vi "PCO_SetFrameRate.vi"(0 "ph":u64, 5 "wFrameRateMode":u16, 7 "dwFrameRate":u32, 9 "dwFrameRateExposure":u32, 11 "error in (no error)":errorcluster {"code" format="%x"}) -> (3 "wFrameRateStatus":u16, 4 "ph out":u64, 6 "ErrorMessage":i32 format="%x", 8 "dwFrameRate out":u32, 10 "dwFrameRateExposure out":u32, 15 "error out":errorcluster {"code" format="%x"})   [LabVIEW 2019, in "SDK.lvlib" / "TimingControl.lvlib"]
doc: "<b>Description:</b>\nThis function does directly set the frame rate and the exposure time of the camera. The frame rate is limited by the readout time and the exposure time.\n\nframe rate <= 1/t_readout frame rate <= 1/t_expos\n\nPlease note that there are some overhead times, therefore the real values can differ slightly, e.g. the maximum frame rate will be a little bit less than 1 / exposure time. The in wFramerateMode parameter defines how the function works if any of the conditions are not met.\n\nIf Recording State is [run] (see PCO_GetRecordingState) the frame rate and exposure time of the camera is changed immediately. The input parameters are adapted according to the given rule in wFramerateMode. The function returns the currently configured frame rate and exposure time.\nIf Recording State of the camera is [stop] the given frame rate and exposure time is stored in the camera. The function does not adapt the input values for frame rate and exposure time. The next call of PCO_ArmCamera validates the input parameters together with other settings. Status of validation can be seen in the returned status wFrameRateStatus.\n\nThe following procedure is recommended:\n. Set PCO_SetRecordingState to [stop]\n. Set frame rate and exposure time using the PCO_SetFrameRate function\n. Do other settings, before or after the PCO_SetFrameRate function\n. Call the PCO_ArmCamera function in order to validate the settings\n. Retrieve the currently set frame rate and exposure time using PCO_GetFrameRate\n\nBecause frame rate and exposure time are also affected by the PCO_SetDelayExposureTime command, it is strongly recommended to use either the PCO_SetFrameRate or the PCO_SetDelayExposureTime command.\n\n<b>Supported camera type:</b>\npco.edge, pco.dimax\n\n<b>Descriptor dependency:</b>\ndwGeneralCapsDESC1: SETFRAMERATE_ENABLED"
uses:
  TimingControl.lvlib
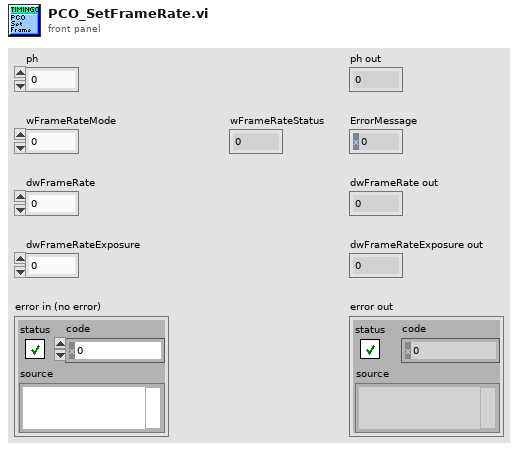
[diagram p1: front panel]
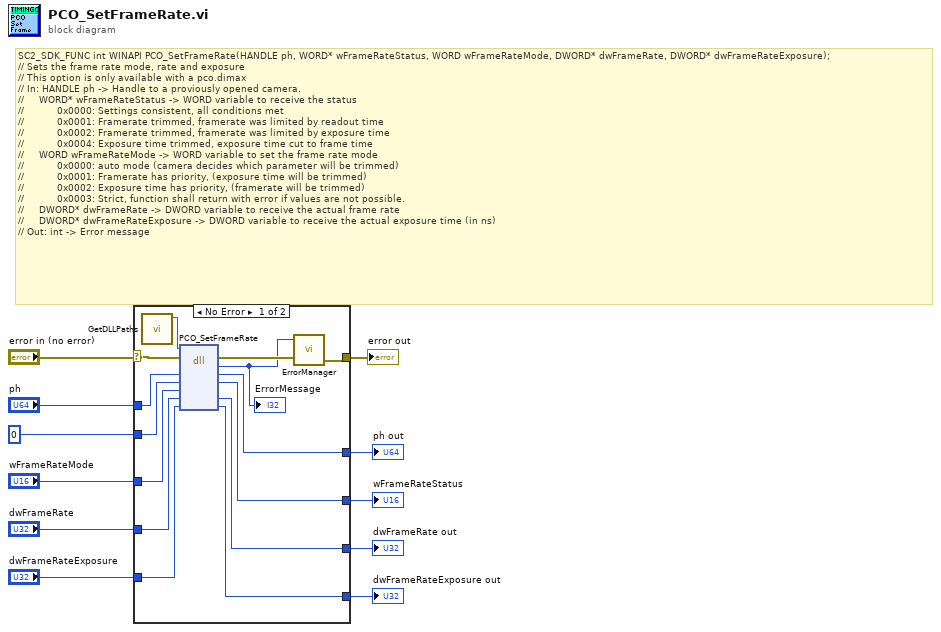
[diagram p0: block diagram]
diagram:
  # "SC2_SDK_FUNC int WINAPI PCO_SetFrameRate(HANDLE ph, WORD* wFrameRateStatus, WORD wFrameRateMode, DWORD* dwFrameRate, DWORD* dwFrameRateExposure);\n// Sets the frame rate mode, rate and exposure\n// This option is only available with a pco.dimax\n// In: HANDLE ph -> Handle to a proviously opened camera.\n//     WORD* wFrameRateStatus -> WORD variable to receive the status\n//           0x0000: Settings consistent, all conditions met\n//           0x0001: Framerate trimmed, framerate was limited by readout time\n//           0x0002: Framerate trimmed, framerate was limited by exposure time\n//           0x0004: Exposure time trimmed, exposure time cut to frame time\n//     WORD wFrameRateMode -> WORD variable to set the frame rate mode\n//           0x0000: auto mode (camera decides which parameter will be trimmed)\n//           0x0001: Framerate has priority, (exposure time will be trimmed)\n//           0x0002: Exposure time has priority, (framerate will be trimmed)\n//           0x0003: Strict, function shall return with error if values are not possible.\n//     DWORD* dwFrameRate -> DWORD variable to receive the actual frame rate\n//     DWORD* dwFrameRateExposure -> DWORD variable to receive the actual exposure time (in ns)\n// Out: int -> Error message"
  n1 = case shown="No Error" "error in (no error)" {
    selector: "error in (no error)" -> [w16 w30]
    tunnel: "ph" -> [w25 w29]
    tunnel: [w24 w29] -> w10
    tunnel: u16 0 ("wFrameRateStatus") -> [w23 w28]
    tunnel: [w22 w28] -> w8
    tunnel: "wFrameRateMode" -> [w21 _]
    tunnel: "dwFrameRate" -> [w20 w27]
    tunnel: [w19 w27] -> w5
    tunnel: "dwFrameRateExposure" -> [w18 w26]
    tunnel: [w17 w26] -> w3
    tunnel: [w14 w30] -> w2
    frame No Error {
      n2 = call "GetDLLPaths.vi"() -> ("SC2_Cam_Path"=w12:path)  [unwired: 8 in, 3 out]
      n3 = dll-call lib="?" fn="PCO_SetFrameRate"(path in=w12, error in=w16, "ph"=w25, "wFrameRateStatus"=w23, "wFrameRateMode"=w21, "dwFrameRate"=w20, "dwFrameRateExposure"=w18) -> (error out=w15:errorcluster, "return type"=w13:i32, "ph"=w24:u64, "wFrameRateStatus"=w22:u16, "dwFrameRate"=w19:u32, "dwFrameRateExposure"=w17:u32)  [unwired: 2 in, 1 out]
      "ErrorMessage" <- w13
      n4 = call "ErrorManager.vi"("error in (no error)"=w15, "error code"=w13) -> ("error out"=w14:errorcluster)  [unwired: 2 in, 1 out]
    }
    frame Error {
    }
  }
  "ph out" <- w10
  "wFrameRateStatus" <- w8
  "dwFrameRate out" <- w5
  "dwFrameRateExposure out" <- w3
  "error out" <- w2
